vi "RSZVL_Init.vi"(8 "error in (no error)":errorcluster {"code" format="%.0x"}, 11 "resource name":string) -> (0 "error out":errorcluster, 3 "VISA resource name out":refnum<visa-resource-name>)   [LabVIEW 2015]
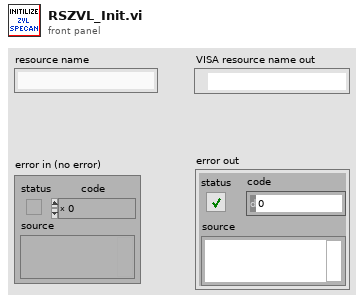
[diagram p1: front panel]
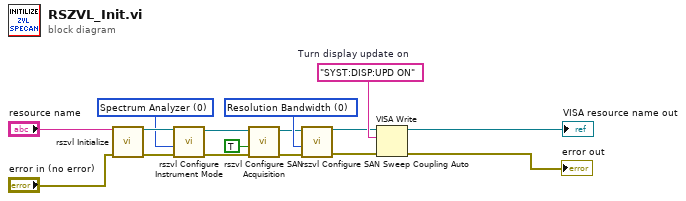
[diagram p0: block diagram]
diagram:
  w10 = 0 items=["Resolution Bandwidth", "Video Bandwidth", "Sweep Time"] ("Sweep Coupling (Resolution Bandwidth)")
  w13 = "SYST:DISP:UPD ON"  # Turn display update on
  w12 = 0 items=["Spectrum Analyzer", "Network Analyzer", "Noise Figure And Gain Measurements", "WCDMA Measurements", "WLAN OFDM Analysis", "WiMAX OFDM/OFDMA Analysis", "Analog Measurement Demodulator", "Bluetooth Measurements", "Cable TV Analyzer"] ("Instrument Mode (Network Analyzer)")
  n1 = call <instrlib>:"rszvl Initialize.vi"("VISA resource name"="resource name", "error in (no error)"="error in (no error)") -> ("VISA resource name out"=w16:refnum<visa-resource-name>, "error out"=w15:errorcluster)  [unwired: 12 in]
  n2 = call <instrlib>:"rszvl Configure Instrument Mode.vi"("error in (no error)"=w15, "Instrument Mode (Network Analyzer)"=w12, "VISA resource name"=w16) -> ("error out"=w5:errorcluster, "VISA resource name out"=w6:refnum<visa-resource-name>)  [unwired: 7 in]
  n3 = call <instrlib>:"rszvl Configure SAN Acquisition.vi"("error in (no error)"=w5, "Sweep Mode Continuous (Off)"=TRUE, "VISA resource name"=w6) -> ("error out"=w9:errorcluster, "VISA resource name out"=w8:refnum<visa-resource-name>)  [unwired: 7 in]
  n4 = call <instrlib>:"rszvl Configure SAN Sweep Coupling Auto.vi"("error in (no error)"=w9, "Sweep Coupling (Resolution Bandwidth)"=w10, "VISA resource name"=w8) -> ("error out"=w3:errorcluster, "VISA resource name out"=w4:refnum<visa-resource-name>)  [unwired: 7 in]
  n5 = VISA Write(VISA resource name=w4, write buffer=w13, error in (no error)=w3) -> (VISA resource name out=→"VISA resource name out":refnum<visa-resource-name>, error out=→"error out":errorcluster)  [unwired: 1 out]
